vi "Align String.vi"(7 "Align Length":i32=20, 10 "String In":string) -> (2 "String Out":string)   [LabVIEW 2024]
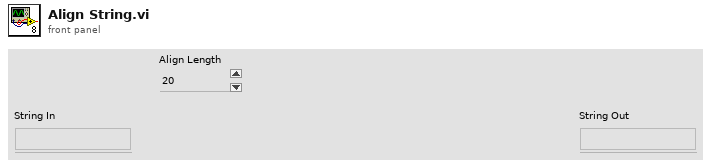
[diagram p1: front panel]
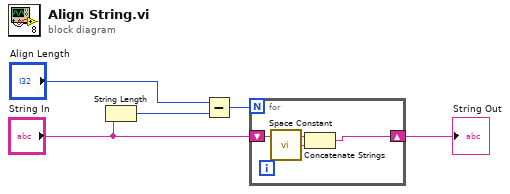
[diagram p0: block diagram]
diagram:
  n1 = String Length(string="String In") -> (length=w4:i32)
  n2 = Subtract(x="Align Length", y=w4) -> (x-y=w3:i32)
  n3 = for {
    N: w3 -> [_]
    shift-right: [w6] -> w1
    shift-left: "String In" -> [w8]
    n4 = call <vilib>:"Space Constant.vi"() -> ("String"=w7:string)
    n5 = Concatenate Strings(w8, w7) -> (w6:string)
  }
  "String Out" <- w1
